vi "Create Value Terminal.vi"(8 "error in (no error)":errorcluster, 9 "Type Descriptor":T1, 11 "VI in":refnum<vi>) -> (0 "error out":errorcluster, 2 "Ctl Refnum":refnum<vi>)   [LabVIEW 2020, in "FlexBlocks.lvlib"]
uses:
  FlexBlocks.lvlib
  Type Descriptor.ctl
  Terminal Direction.ctl
  Value Mode.ctl
  Special Terminal.ctl
  <vilib>/Utility/miscctls.llb/LVPointTypeDef.ctl
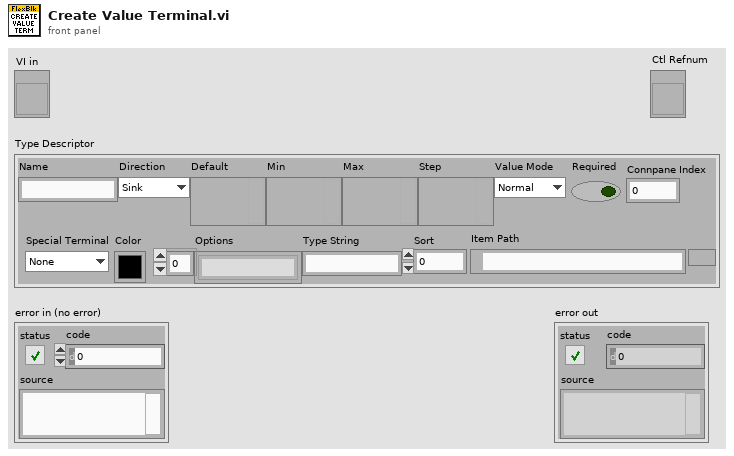
[diagram p1: front panel]
types:
  T1 = typedef "FlexBlocks.lvlib/Type Descriptor.ctl" = cluster{"Name":string, "Direction":T2, "Default":variant, "Min":variant, "Max":variant, "Step":variant, "Value Mode":T3, "Required":bool, "Connpane Index":i32, "Special Terminal":T4, "Color":u32, "Options":string[], "Type String":string, "Sort":i32, "Item Path":path}
  T2 = typedef "FlexBlocks.lvlib/Terminal Direction.ctl" = enum16{"Sink", "Source"}
  T3 = typedef "FlexBlocks.lvlib/Value Mode.ctl" = enum16{"Normal", "Range", "Select"}
  T4 = typedef "FlexBlocks.lvlib/Special Terminal.ctl" = enum16{"None", "Action", "Init", "Tag", "State in", "State out", "Error"}
  T5 = typedef "LVPointTypeDef.ctl" = cluster{"Horizontal":i16, "Vertical":i16}
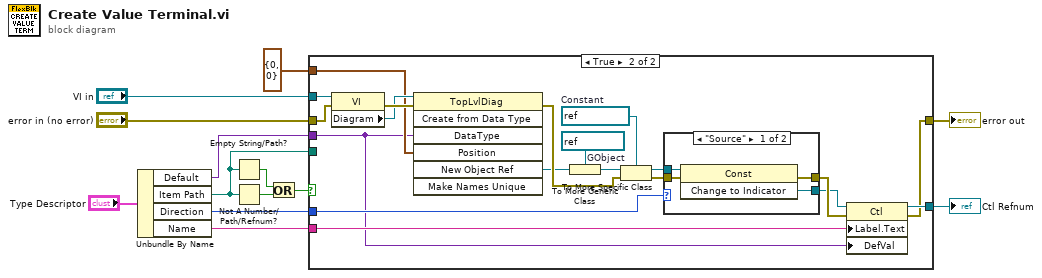
[diagram p0: block diagram]
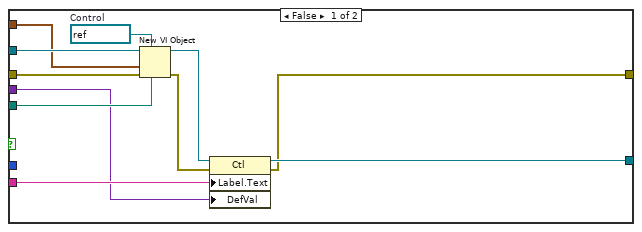
[diagram p2: hidden frame]
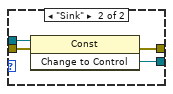
[diagram p3: hidden frame]
diagram:
  n1 = Unbundle By Name("Type Descriptor") -> ("Default"=w13:variant, "Item Path"=w9:path, "Direction"=w7:T2, "Name"=w1:string)
  n2 = Empty String/Path?(string/path=w9) -> (empty?=w12:bool)
  n3 = Not A Number/Path/Refnum?(number/path/refnum=w9) -> (NaN/Path/Refnum?=w11:bool)
  n4 = Or(x=w12, y=w11) -> (x .or. y?=w10:bool)
  n5 = case shown="True" w10 {
    tunnel: [w14 w25] -> w5
    tunnel: w13 -> [w16 w27]
    tunnel: [w19 w26] -> w6
    tunnel: w7 -> [_ w35]
    tunnel: w9 -> [w24 _]
    tunnel: "VI in" -> [w22 w34]
    tunnel: "error in (no error)" -> [w21 w33]
    tunnel: T5 {"Horizontal"=0, "Vertical"=0} ("location") -> [w20 w30]
    tunnel: w1 -> [w17 w28]
    frame False {
      w23 = refnum<vi> refnum  # Control
      n6 = New VI Object(vi object class=w23, owner refnum=w22, position/next to=w20, 6:w24, 8:w21) -> (object refnum=w18:refnum<vi>, 0:w15:errorcluster)  [unwired: 3 in]
      n7 = property class="Ctl"(reference=w18, error in=w15, "Label.Text"=w17, "DefVal"=w16) -> (reference out=w19:refnum<vi>, error out=w14:errorcluster)
    }
    frame True {
      w38 = refnum<vi> refnum  # Constant
      w40 = refnum<vi> refnum  # GObject
      n8 = property class="VI"(reference=w34, error in=w33) -> (error out=w32:errorcluster, "Diagram"=w31:refnum<vi>)  [unwired: 1 out]
      n9 = invoke class="TopLvlDiag" method="Create from Data Type"(reference=w31, error in=w32, "DataType"=w27, "Position"=w30) -> (error out=w42:errorcluster, "New Object Ref"=w41:refnum<vi>)  [unwired: 3 in, 5 out]
      n10 = To More Generic Class(target class=w40, reference=w41) -> (generic class reference=w39:refnum<vi>)
      n11 = To More Specific Class(target class=w38, reference=w39, error in=w42) -> (specific class reference=w37:refnum<vi>, error out=w36:errorcluster)
      n12 = case shown="\"Source\"" w35 {
        tunnel: [w45 w51] -> w43
        tunnel: w37 -> [w47 w50]
        tunnel: w36 -> [w46 w49]
        tunnel: [w44 w48] -> w29
        frame "Source" {
          n13 = invoke class="Const" method="Change to Indicator"(reference=w47, error in=w46) -> (error out=w45:errorcluster, "Change to Indicator"=w44:refnum<vi>)  [unwired: 1 in, 1 out]
        }
        frame "Sink" {
          n14 = invoke class="Const" method="Change to Control"(reference=w50, error in=w49) -> (error out=w51:errorcluster, "Change to Control"=w48:refnum<vi>)  [unwired: 1 in, 1 out]
        }
      }
      n15 = property class="Ctl"(reference=w29, error in=w43, "Label.Text"=w28, "DefVal"=w27) -> (reference out=w26:refnum<vi>, error out=w25:errorcluster)
    }
  }
  "Ctl Refnum" <- w6
  "error out" <- w5
